vi "2Words2Float.vi"(1 "input":u16[](array[numeric])) -> (0 "value":sgl)   [LabVIEW 2020, in "SMCD14_lib.lvlib"]
uses:
  SMCD14_lib.lvlib
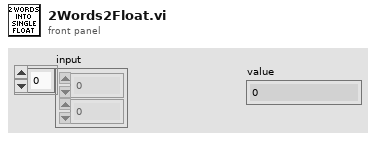
[diagram p1: front panel]
types:
  T1 = enum16{"big-endian, network order", "native, host order", "little-endian"}
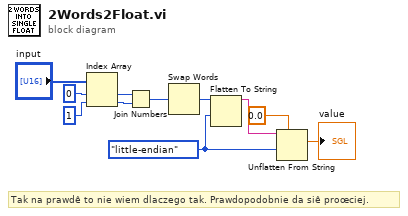
[diagram p0: block diagram]
diagram:
  w3 = T1."little-endian" ("byte order (0:big-endian, network order)")
  # "Tak na prawdê to nie wiem dlaczego tak. Prawdopodobnie da siê proœciej."
  n1 = Index Array(array="input", index #1=0 ("index"), index #2=1 ("index")) -> (element #1=w8:u16, element #2=w7:u16)
  n2 = Join Numbers(hi=w8, lo=w7) -> ((hi.lo)=w6:u32)
  n3 = Swap Words(1:w6) -> (0:w4:u32)
  n4 = Flatten To String(anything=w4, byte order (0:big-endian, network order)=w3) -> (data string=w5:string)  [unwired: 2 in, 2 out]
  n5 = Unflatten From String(type=sgl 0.0, binary string=w5, byte order (0:big-endian, network order)=w3) -> (value=→"value":sgl)  [unwired: 2 in, 2 out]
